vi "dsmmTrackNeuron.vi"(0 "index in reference brain":i32, 7 "reference brain":dbl[][](array[numeric]), 11 "current brain":dbl[][](array[numeric]), 12 "beta":dbl=1.0 format="%#_13g", 13 "lambda":dbl=5.0 format="%#_13g", 14 "gamma0":dbl=0.1 format="%#_13g") -> (4 "position in current brain":dbl[](array[numeric]))   [LabVIEW 2017]
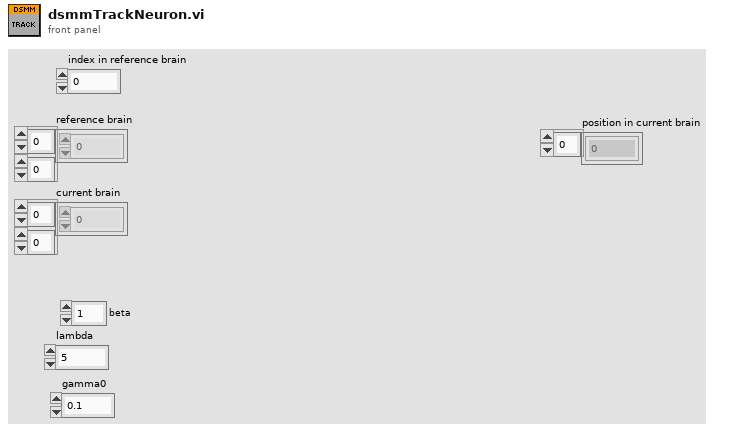
[diagram p1: front panel]
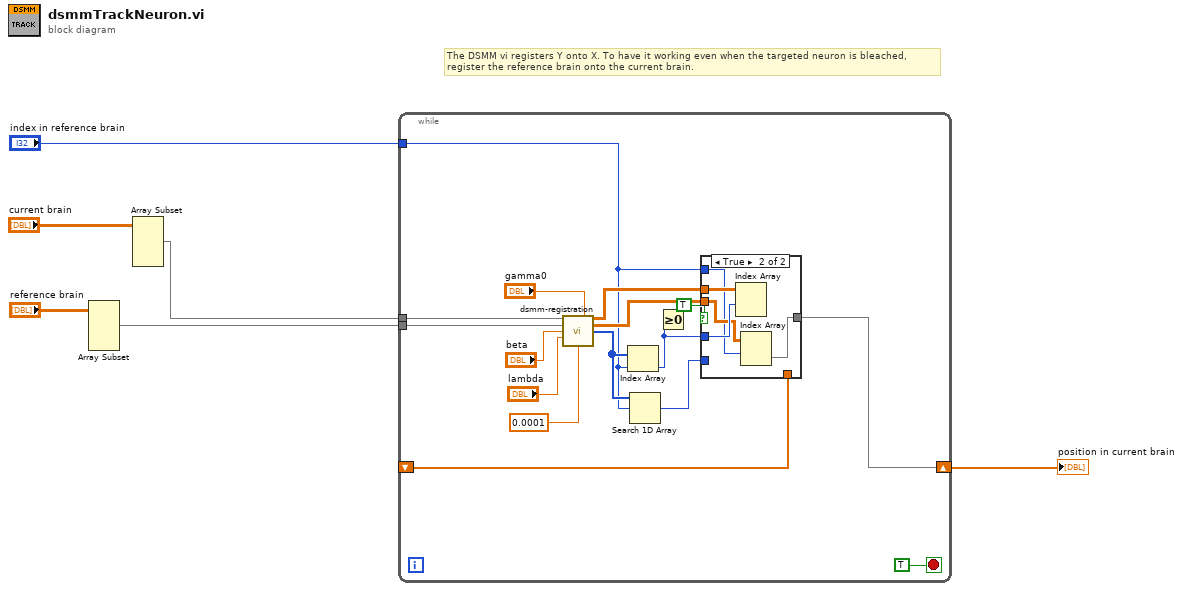
[diagram p0: block diagram]
diagram:
  # "The DSMM vi registers Y onto X. To have it working even when the targeted neuron is bleached,\nregister the reference brain onto the current brain."
  n1 = Array Subset(array="reference brain") -> (w5:dbl[][])  [unwired: 4 in]
  n2 = Array Subset(array="current brain") -> (w6:dbl[][])  [unwired: 4 in]
  n3 = while {
    tunnel: w6 -> [w18]
    tunnel: w5 -> [w17]
    tunnel: "index in reference brain" -> [w11]
    shift-right: [w10] -> w1
    shift-left: _ -> [w8]
    stop <- TRUE stop-if-true
    n4 = call "dsmm-registration.vi"("X"=w18, "gamma0"="gamma0", "Y"=w17, "beta"="beta", "lambda"="lambda", "conv_epsilon"=0.0001) -> ("X out"=w15:dbl[][], "Y out"=w16:dbl[][], "Match"=w14:i32[])  [unwired: 6 in, 1 out]
    n5 = Index Array(array=w14, index=w11) -> (element=w12:i32)
    n6 = Search 1D Array(1D array=w14, element=w11) -> (index of element=w13:i32)  [unwired: 1 in]
    n7 = Greater Or Equal To 0?(x=w12) -> ()  [unwired: 1 out]
    n8 = case shown="True" TRUE {
      tunnel: w16 -> [_ w26]
      tunnel: [w23 w24] -> w10
      tunnel: w8 -> [w23 _]
      tunnel: w11 -> [_ w25]
      tunnel: w15 -> [_ w28]
      tunnel: w13 -> [_ _]
      tunnel: w12 -> [_ w27]
      frame False {
      }
      frame True {
        n9 = Index Array(array=w28, index (row)=w27) -> ()  [unwired: 1 in, 1 out]
        n10 = Index Array(array=w26, index (row)=w25) -> (element=w24:dbl[])  [unwired: 1 in]
      }
    }
  }
  "position in current brain" <- w1
